vi "SinWaveGenerate 1.vi"() -> ()   [LabVIEW 2020]
uses:
  <vilib>/Utility/miscctls.llb/LVDateTimeRec.ctl
  <vilib>/Utility/miscctls.llb/LVAnnotationListTypeDef.ctl
  <vilib>/Waveform/WDTOps.llb/WDT Append Waveforms DBL.vi
  <vilib>/Waveform/WDTOps.llb/WDT Get Waveform Time Array DBL.vi
  <vilib>/measure/NI_MABase.lvlib
panel:
  in  "Kaydet":bool
  in  "Tabloları sil":bool
  in  "Oluştur":bool
  in  "Sinyaller arasını rampa ile birleştir":bool
  in  "Sin Fonksiyonları Arasındaki Düzeltme Artış Miktarı Amp":dbl=50.0 format="%#_13g"
  in  "Tab Control":T1(tab)
  out "Datada kullanılan sinyaller":waveform(dbl)[](graph)
  out "Sinyaller arasındaki geçiş kN farkı":cluster{i32[], "Y":dbl[]}[](graph)
  out "Sinyal Önizleme":waveform(dbl)(graph)
  out "Sinyal Önizleme":waveform(dbl)(graph)
  in  "stop":bool
  in  "Sin wave generate":T2(array[cluster])=[{"Örnekleme Ayarları"={"Fs"=100.0, "#s"=100.0}, "Sinyal Ayarları"={"Frekans"=1.0, "Faz"=0.0, "Genlik"=16.75, "Offset"=0.65, "Cycle"=6.0, "signal type"=enum."Sine Wave"}, "Amp Ratio"=1.0, "Toplam Tekrar"=1.0}, {"Örnekleme Ayarları"={"Fs"=100.0, "#s"=100.0}, "Sinyal Ayarları"={"Frekans"=1.0, "Faz"=0.0, "Genlik"=4.2, "Offset"=0.1, "Cycle"=1.0, "signal type"=enum."Sine Wave"}, "Amp Ratio"=1.0, "Toplam Tekrar"=9.0}, {"Örnekleme Ayarları"={"Fs"=100.0, "#s"=100.0}, "Sinyal Ayarları"={"Frekans"=1.0, "Faz"=0.0, "Genlik"=6.0, "Offset"=0.1, "Cycle"=1.0, "signal type"=enum."Sine Wave"}, "Amp Ratio"=1.0, "Toplam Tekrar"=50.0}, {"Örnekleme Ayarları"={"Fs"=100.0, "#s"=100.0}, "Sinyal Ayarları"={"Frekans"=1.0, "Faz"=0.0, "Genlik"=20.05, "Offset"=-7.45, "Cycle"=1.0, "signal type"=enum."Sine Wave"}, "Amp Ratio"=1.0, "Toplam Tekrar"=1.0}] {"Amp Ratio" format="%.2p"; "Sinyal Ayarları"."Faz" format="%.2p"; "Sinyal Ayarları"."Frekans" format="%0.2p"; "Örnekleme Ayarları"."Fs" format="%.2p"}
  # "Offset"
  # "Amplitude"
  # "Level 4"
  # "16,75"
  # "+0,65"
  # "Level 3"
  # "4,2"
  # "+0,1"
  # "Level 2"
  # "6,0"
  # "+0,1"
  # "Level 1"
  # "20,05"
  # "-7,45"
  # "array 0"
  # "array 1"
  # "array 2"
  # "array 3"
  # "((((((6xLevel 4)+level3)x9 )+ level2)x50)+ level1) x 200"
  # "(((Cycle*sinyal)*Toplam Tekrar + ......(Array n Cycle*Array n sinyal) * Array n Toplam Tekrar)))"
  # "Array 0 =>"
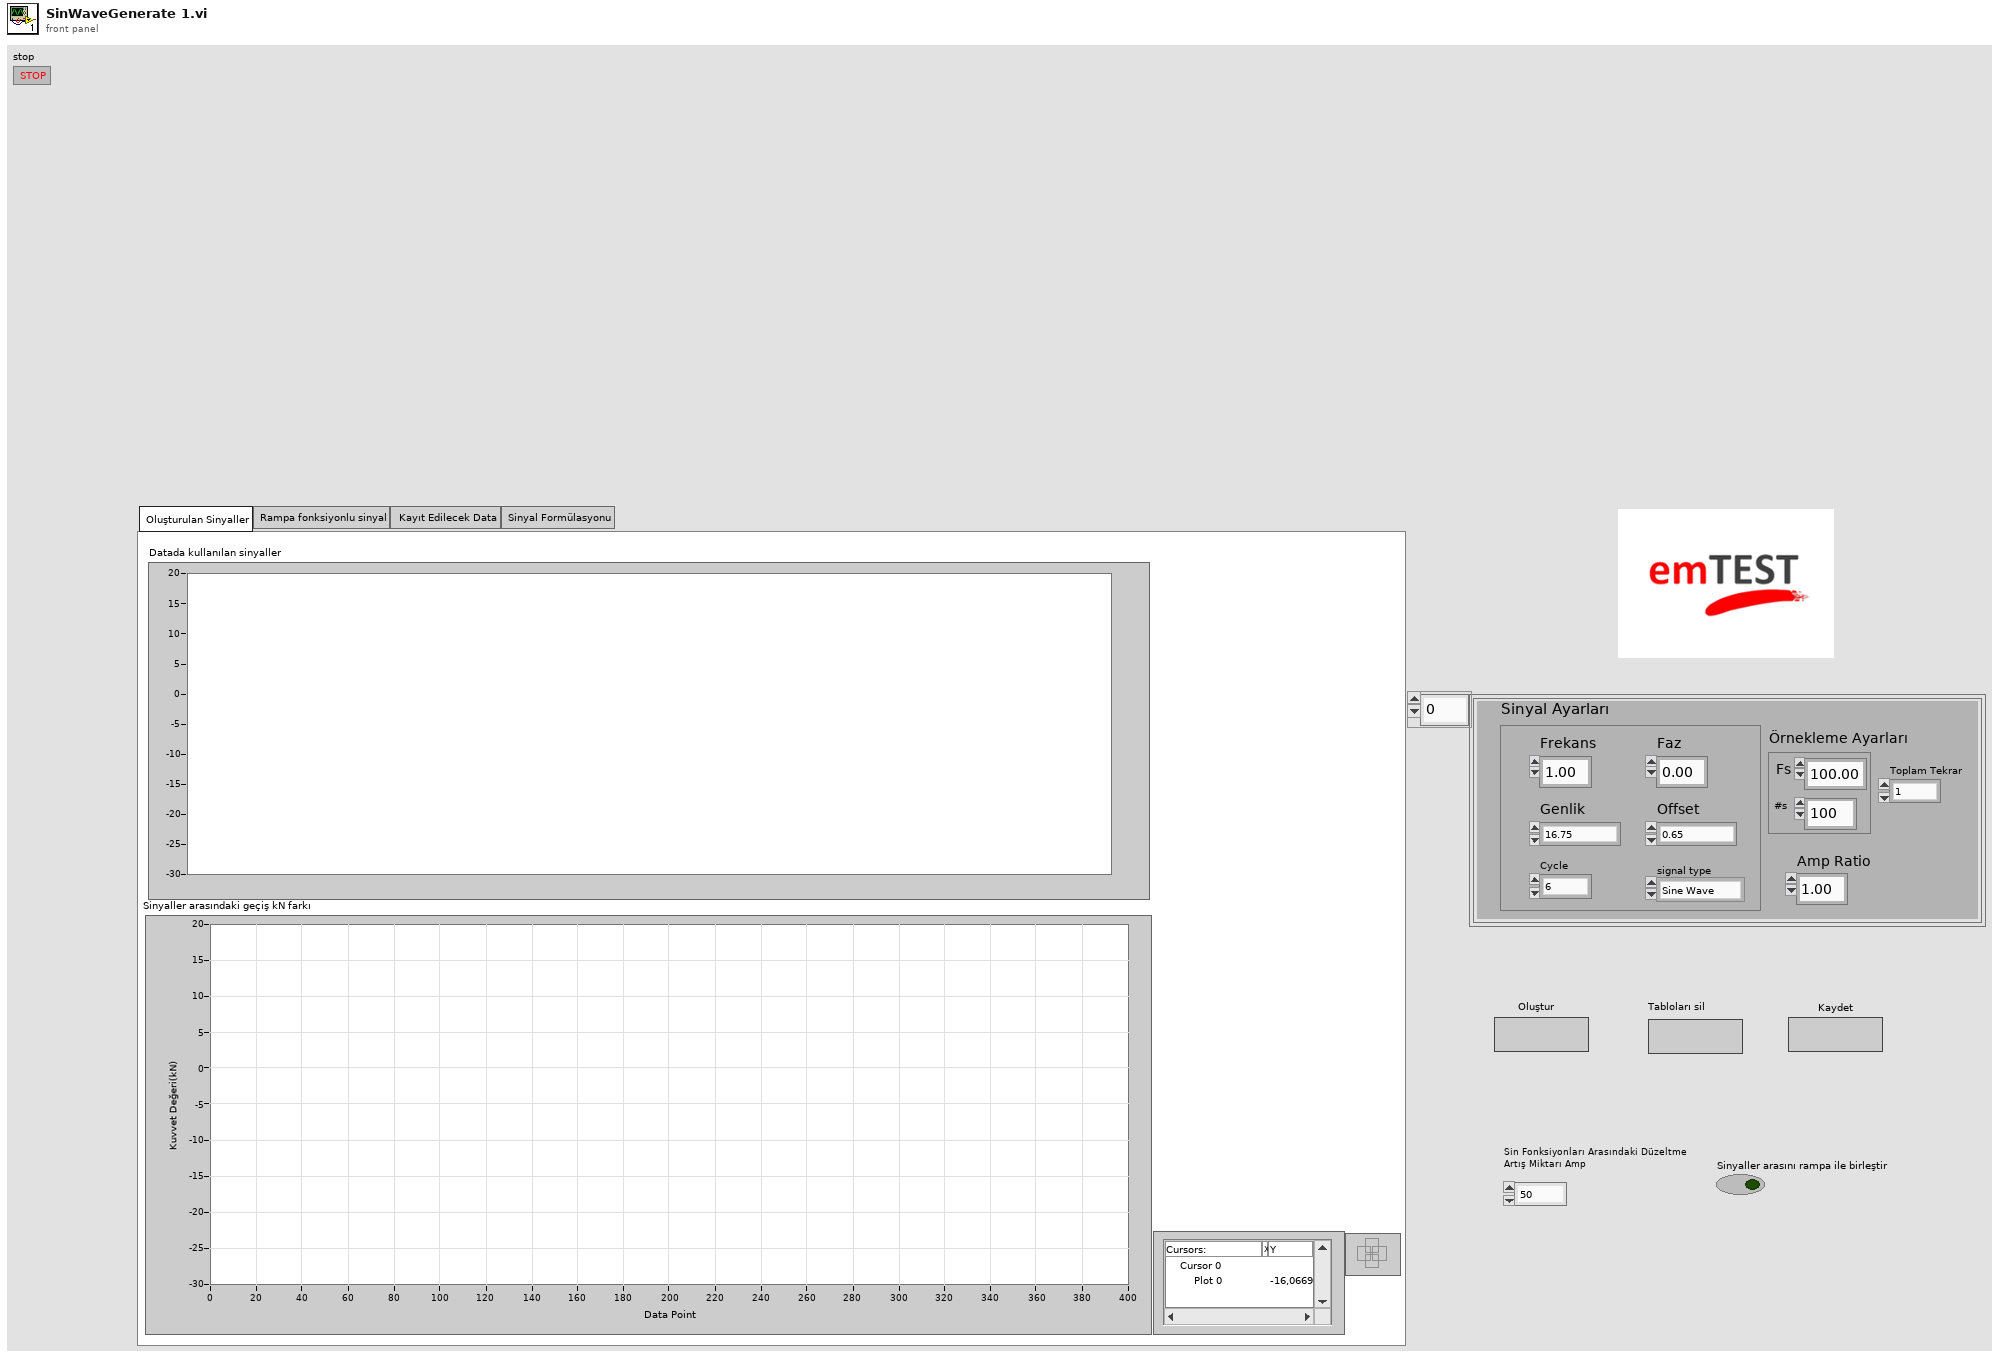
[diagram p1: front panel]
types:
  T1 = enum32{"Oluşturulan Sinyaller", "Rampa fonksiyonlu sinyal", "Kayıt Edilecek Data ", "Sinyal Formülasyonu"}
  T2 = cluster{"Örnekleme Ayarları":cluster{"Fs":dbl, "#s":dbl}, "Sinyal Ayarları":cluster{"Frekans":dbl, "Faz":dbl, "Genlik":dbl, "Offset":dbl, "Cycle":dbl, "signal type":enum16{"Sine Wave", "Triangle Wave", "Square Wave", "Sawtooth Wave"}}, "Amp Ratio":dbl, "Toplam Tekrar":dbl}[]
  T3 = enum16{"open", "replace", "create", "open or create", "replace or create", "replace or create with confirmation"}
  T4 = typedef "LVDateTimeRec.ctl" = cluster{"fractional second":dbl, "second":i32, "minute":i32, "hour":i32, "day of month":i32, "month":i32, "year":i32, "day of week":i32, "day of year":i32, "DST":i32}
  T5 = cluster{"Name":string, "Color":u32, "Style":u8, "Point Style":u8, "Name Visible":bool, "Allow Drag":bool, "Annotation Mode":u32, "Plot":i32, "Index":i32, "Position":cluster{"X":dbl, "Y":dbl}, "X Scale":u32, "Y Scale":u32, "Show Arrow":bool, "Lock Name":bool, "Plot Area":i32, "Label Offset":cluster{"X":dbl, "Y":dbl}}
  T6 = typedef "LVAnnotationListTypeDef.ctl" = cluster{"Name":string, "Color":u32, "Style":u8, "Point Style":u8, "Name Visible":bool, "Allow Drag":bool, "Annotation Mode":u32, "Plot":i32, "Index":i32, "Position":cluster{"X":dbl, "Y":dbl}, "X Scale":u32, "Y Scale":u32, "Show Arrow":bool, "Lock Name":bool, "Plot Area":i32, "Label Offset":cluster{"X":dbl, "Y":dbl}}[]
  T7 = enum16{"Sine Wave", "Triangle Wave", "Square Wave", "Sawtooth Wave"}
  T8 = cluster{"Frekans":dbl, "Faz":dbl, "Genlik":dbl, "Offset":dbl, "Cycle":dbl, "signal type":enum16{"Sine Wave", "Triangle Wave", "Square Wave", "Sawtooth Wave"}}
  T9 = cluster{"Name":string, "Color":u32, "Style":u8, "Point Style":u8, "Name Visible":bool, "Allow Drag":bool, "Annotation Mode":u32, "Plot":i32, "Index":i32, "Position":cluster{"X":dbl, "Y":dbl}, "X Scale":u32, "Y Scale":u32, "Show Arrow":bool, "Lock Name":bool, "Plot Area":i32, "Label Offset":cluster{"X":dbl, "Y":dbl}}[]
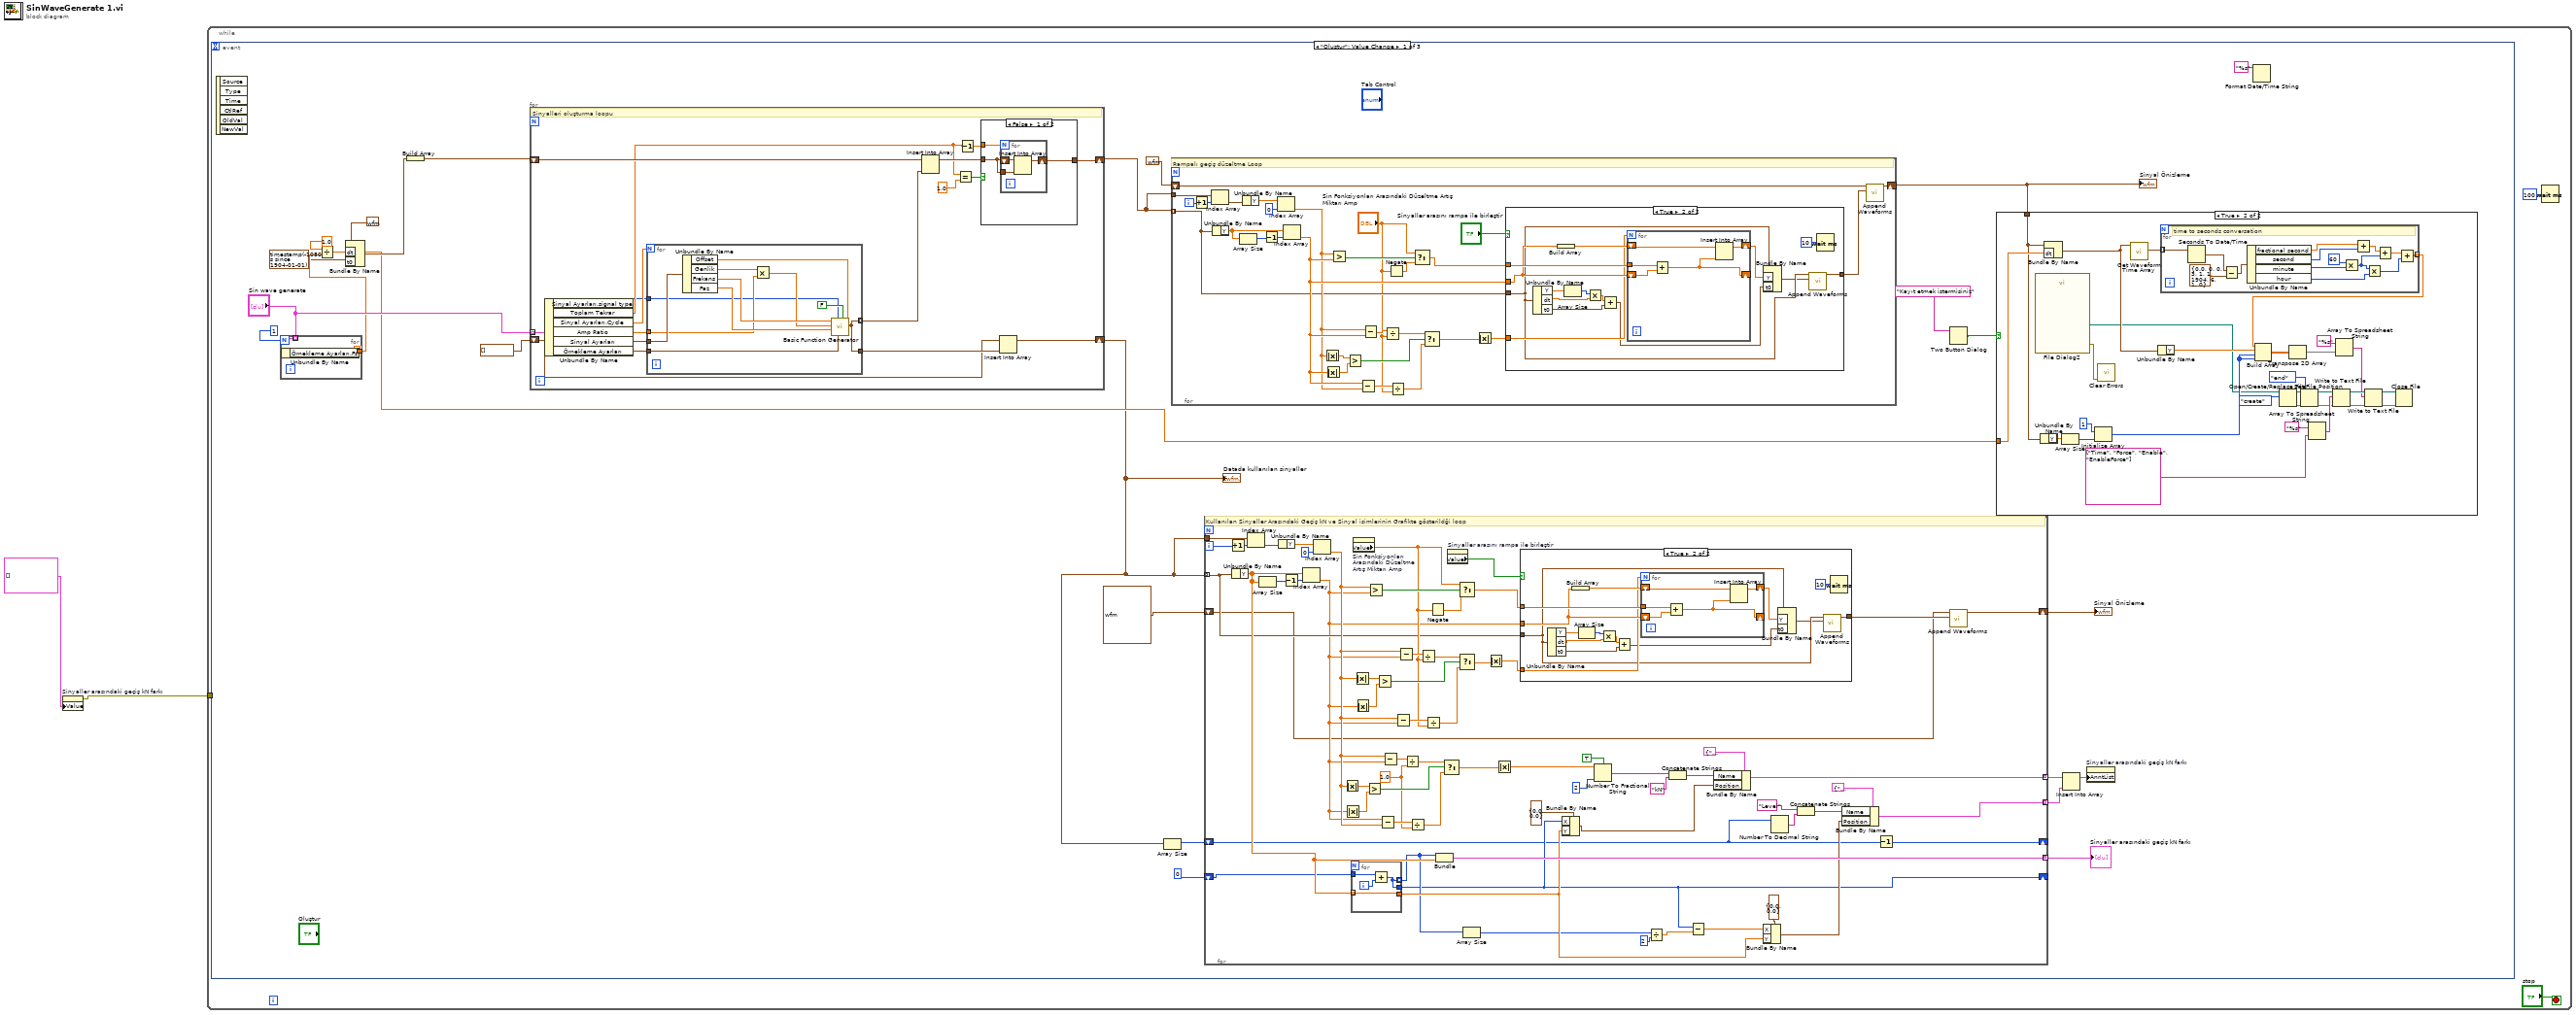
[diagram p0: block diagram]
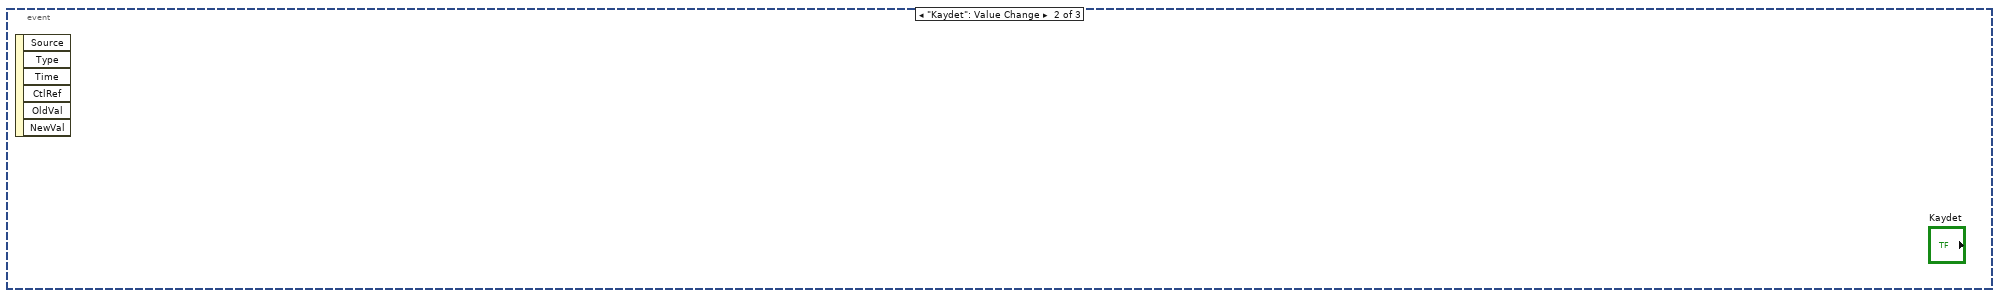
[diagram p6: hidden frame]
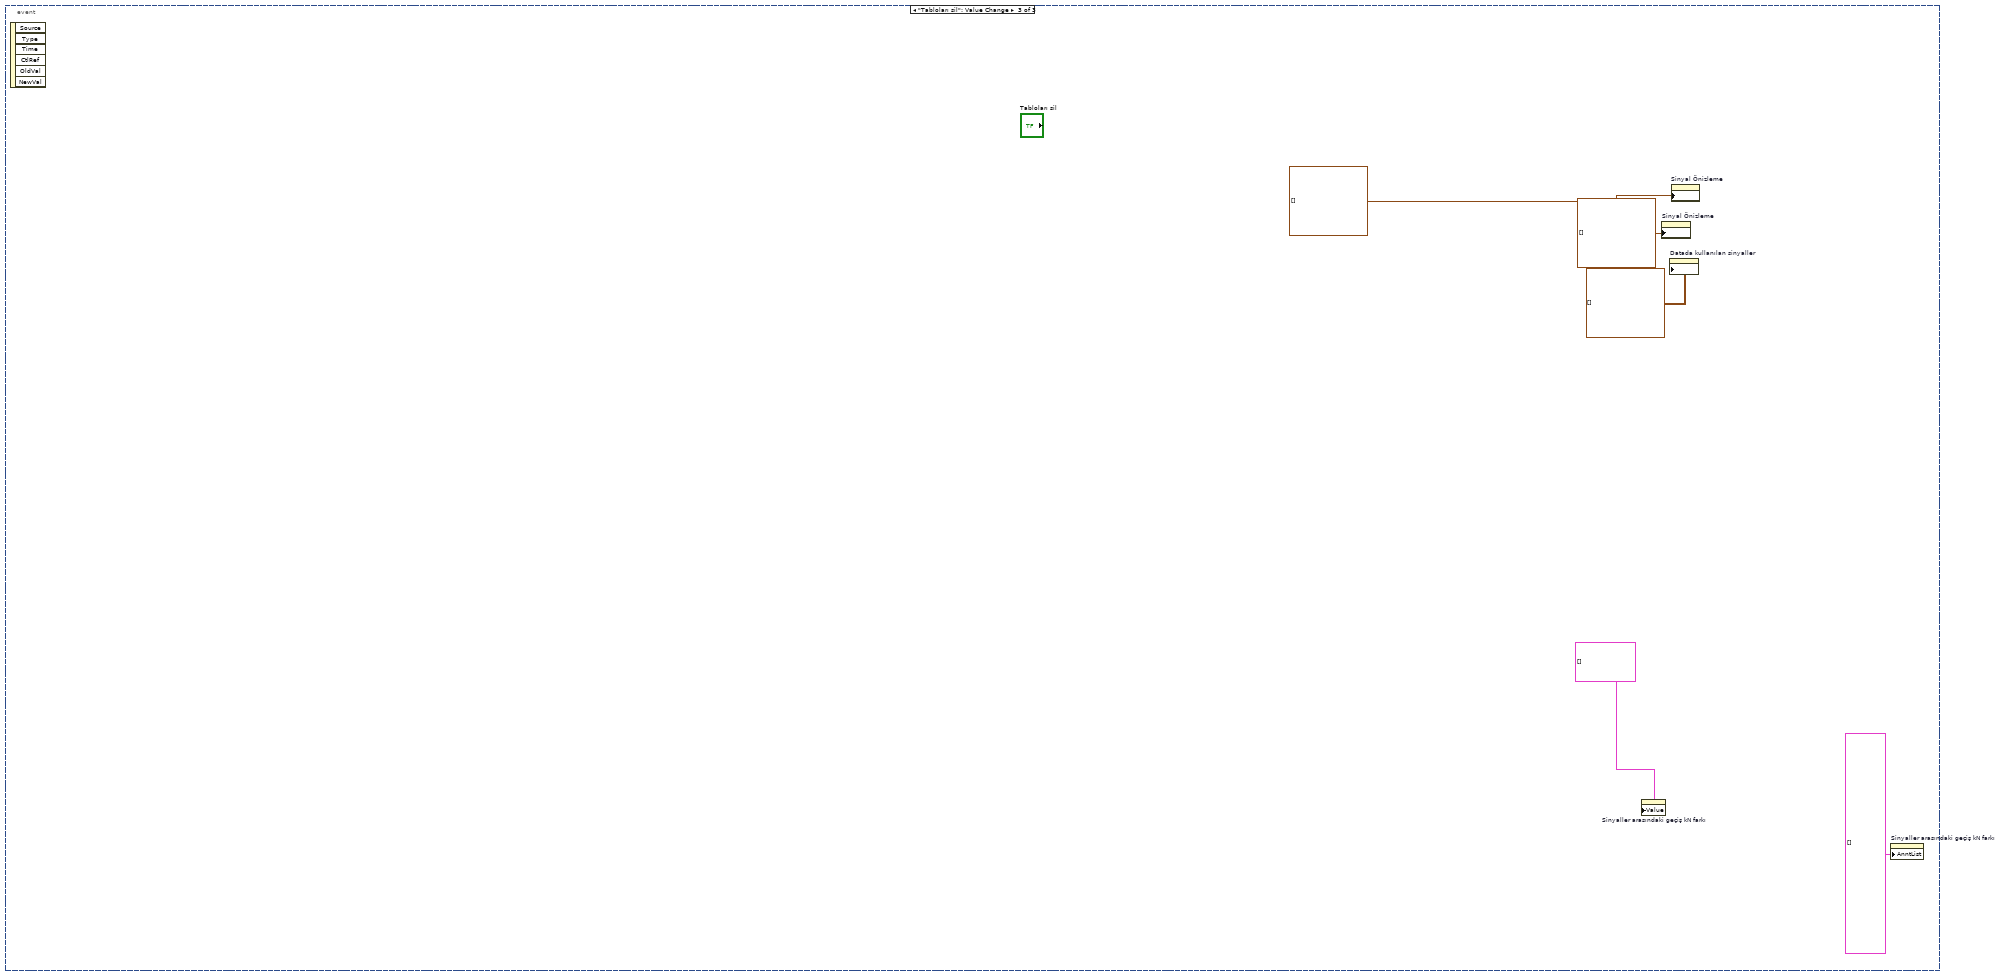
[diagram p7: hidden frame]
diagram:
  n1 = property on="Sinyaller arasındaki geçiş kN farkı" class="XYGraph (strict)"("Value"=cluster{i32[], "Y":dbl[]}[] [] ("XY Graph")) -> (error out=w1:errorcluster)  [unwired: 2 in, 1 out]
  n2 = while {
    tunnel: w1 -> [_]
    stop <- "stop" stop-if-true
    n3 = event shown="[0] \"Oluştur\": Value Change" {
      selector: _ -> [_ _ _]
      dyn-events: _ -> [_ _ _]
      timeout: _ -> [_ _ _]
      event "Oluştur": Value Change {
        n4 = event-data() -> ()  [unwired: 1 in, 6 out]
        n5 = for {
          N: 1 -> [_]
          tunnel: "Sin wave generate" -> [w215] mode=indexing
          tunnel: [w214] -> w25
          n6 = Unbundle By Name(w215) -> ("Örnekleme Ayarları.Fs"=w214:dbl)
        }
        n7 = Divide(x=1.0, y=w25) -> (x/y=w20:dbl)
        n8 = Bundle By Name(cluster=waveform(dbl) {"t0"=timestamp(0 s since 1904-01-01), "dt"=1.0, "Y"=[]} ("signal out"), "dt"=w20, "t0"=timestamp(-10800 s since 1904-01-01)) -> (w23:waveform(dbl))
        n9 = Build Array(w23) -> (w22:waveform(dbl)[])
        n10 = for {
          tunnel: "Sin wave generate" -> [w231] mode=indexing
          shift-right: [w224] -> w19
          shift-left: w22 -> [w230]
          shift-right: [w218] -> w6
          shift-left: waveform(dbl)[] [] -> [w217]
          # "Sinyalleri oluşturma loopu"
          n11 = Unbundle By Name(w231) -> ("Sinyal Ayarları.signal type"=w216:T7, "Toplam Tekrar"=w221:dbl, "Sinyal Ayarları.Cycle"=w227:dbl, "Amp Ratio"=w229:dbl, "Sinyal Ayarları"=w232:T8, "Örnekleme Ayarları"=w228:cluster{"Fs":dbl, "#s":dbl})
          n12 = for {
            N: w227 -> [_]
            tunnel: w232 -> [w248]
            tunnel: w229 -> [w246]
            tunnel: w228 -> [w243]
            tunnel: [w241] -> w226 mode=indexing
            tunnel: [w241] -> w219
            tunnel: w216 -> [w240]
            n13 = Unbundle By Name(w248) -> ("Offset"=w244:dbl, "Genlik"=w247:dbl, "Frekans"=w250:dbl, "Faz"=w249:dbl)
            n14 = Multiply(x=w247, y=w246) -> (x*y=w245:dbl)
            n15 = call <vilib>:"Basic Function Generator.vi"("offset"=w244, "reset signal"=FALSE, "sampling info"=w243, "signal type"=w240, "phase"=w249, "amplitude"=w245, "frequency"=w250) -> ("signal out"=w241:waveform(dbl))  [unwired: 2 in, 2 out]
          }
          n16 = Insert Into Array(array=w230, new element=w226) -> (w225:waveform(dbl)[])  [unwired: 1 in]
          n17 = Equal?(x=w221, y=1.0) -> (x = y?=w222:bool)
          n18 = Decrement(x=w221) -> (x-1=w220:dbl)
          n19 = case shown="False" w222 {
            tunnel: w225 -> [w235 w239]
            tunnel: w220 -> [w234 _]
            tunnel: [w233 w239] -> w224
            frame False {
              n20 = for {
                N: w234 -> [_]
                shift-right: [w237] -> w233
                shift-left: w235 -> [w238]
                tunnel: w235 -> [w236]
                n21 = Insert Into Array(array=w238, new element=w236) -> (w237:waveform(dbl)[])  [unwired: 1 in]
              }
            }
            frame True {
            }
          }
          n22 = Insert Into Array(array=w217, new element=w219) -> (w218:waveform(dbl)[])  [unwired: 1 in]
        }
        "Datada kullanılan sinyaller" <- w6
        n23 = Array Size(array=w6) -> (size(s)=w5:i32)
        n24 = for {
          tunnel: w19 -> [w170] mode=indexing
          tunnel: w19 -> [w189]
          shift-right: [w168] -> w14
          shift-left: waveform(dbl) {"t0"=timestamp(0 s since 1904-01-01), "dt"=1.0, "Y"=[]} ("waveform out") -> [w167]
          i -> [w188]
          # "Rampalı geçiş düzeltme Loop"
          n25 = Increment(x=w188) -> (x+1=w187:i32)
          n26 = Index Array(array=w189, index=w187) -> (element=w186:waveform(dbl))
          n27 = Unbundle By Name(w170) -> ("Y"=w190:dbl[])
          n28 = Array Size(array=w190) -> (size(s)=w191:i32)
          n29 = Unbundle By Name(w186) -> ("Y"=w185:dbl[])
          n30 = Decrement(x=w191) -> (x-1=w192:i32)
          n31 = Index Array(array=w185, index=0) -> (element=w175:dbl)
          n32 = Index Array(array=w190, index=w192) -> (element=w176:dbl)
          n33 = Absolute Value(x=w175) -> (abs(x)=w181:dbl)
          n34 = Absolute Value(x=w176) -> (abs(x)=w180:dbl)
          n35 = Greater?(x=w175, y=w176) -> (0:w182:bool)
          n36 = Greater?(x=w181, y=w180) -> (0:w179:bool)
          n37 = Subtract(x=w176, y=w175) -> (x-y=w174:dbl)
          n38 = Subtract(x=w175, y=w176) -> (x-y=w178:dbl)
          n39 = Divide(x=w178, y="Sin Fonksiyonları Arasındaki Düzeltme Artış Miktarı Amp") -> (x/y=w177:dbl)
          n40 = Negate(x="Sin Fonksiyonları Arasındaki Düzeltme Artış Miktarı Amp") -> (-x=w166:dbl)
          n41 = Divide(x=w174, y="Sin Fonksiyonları Arasındaki Düzeltme Artış Miktarı Amp") -> (x/y=w173:dbl)
          n42 = Select(t="Sin Fonksiyonları Arasındaki Düzeltme Artış Miktarı Amp", s=w182, f=w166) -> (s? t:f=w183:dbl)
          n43 = Select(t=w177, s=w179, f=w173) -> (s? t:f=w172:dbl)
          n44 = Absolute Value(x=w172) -> (abs(x)=w171:dbl)
          n45 = case shown="True" "Sinyaller arasını rampa ile birleştir" {
            tunnel: w170 -> [w193 w196]
            tunnel: w176 -> [_ w207]
            tunnel: w183 -> [_ w208]
            tunnel: [w193 w197] -> w169
            tunnel: w171 -> [_ w204]
            frame False {
            }
            frame True {
              n46 = Unbundle By Name(w196) -> ("Y"=w203:dbl[], "dt"=w198:dbl, "t0"=w200:timestamp)
              n47 = Build Array(w207) -> (w206:dbl[])
              n48 = Array Size(array=w203) -> (size(s)=w202:i32)
              n49 = Multiply(x=w202, y=w198) -> (x*y=w201:dbl)
              n50 = Add(x=w201, y=w200) -> (x+y=w199:timestamp)
              n51 = for {
                N: w204 -> [_]
                tunnel: w208 -> [w213]
                shift-right: [w209] -> _
                shift-left: w207 -> [w212]
                shift-right: [w211] -> w205
                shift-left: w206 -> [w210]
                n52 = Add(x=w213, y=w212) -> (x+y=w209:dbl)
                n53 = Insert Into Array(array=w210, new element=w209) -> (w211:dbl[])  [unwired: 1 in]
              }
              n54 = Bundle By Name(cluster=w196, "Y"=w205, "t0"=w199) -> (w195:waveform(dbl))
              n55 = call-poly <vilib>:"Append Waveforms.vi"("waveform B"=w195, "waveform A"=w196) -> ("waveform out"=w197:waveform(dbl))  [unwired: 8 in, 1 out]
              n56 = Wait (ms)(milliseconds to wait=u32 10) -> ()  [unwired: 1 out]
            }
          }
          n57 = call-poly <vilib>:"Append Waveforms.vi"("waveform B"=w169, "waveform A"=w167) -> ("waveform out"=w168:waveform(dbl))  [unwired: 8 in, 1 out]
        }
        "Sinyal Önizleme" <- w14
        n58 = for {
          tunnel: w6 -> [w100] mode=indexing
          tunnel: w6 -> [w136]
          shift-right: [w79] -> _
          shift-left: 0 -> [w76]
          tunnel: [w121] -> w17 mode=indexing
          tunnel: [w120] -> w9 mode=indexing
          shift-right: [w95] -> w16
          shift-left: waveform(dbl) {"t0"=timestamp(0 s since 1904-01-01), "dt"=1.0, "Y"=[]} -> [w94]
          tunnel: [w82] -> w8 mode=indexing
          shift-right: [w74] -> _
          shift-left: w5 -> [w73]
          i -> [w135]
          w119 = 1.0 ("y")
          # "Kullanılan Sinyaller Arasındaki Geçiş kN ve Sinyal isimlerinin Grafikte gösterildği loop"
          n59 = Increment(x=w135) -> (x+1=w134:i32)
          n60 = Unbundle By Name(w100) -> ("Y"=w122:dbl[])
          n61 = Index Array(array=w136, index=w134) -> (element=w133:waveform(dbl))
          n62 = Array Size(array=w122) -> (size(s)=w137:i32)
          n63 = Unbundle By Name(w133) -> ("Y"=w132:dbl[])
          n64 = Decrement(x=w137) -> (x-1=w138:i32)
          n65 = Index Array(array=w122, index=w138) -> (element=w99:dbl)
          n66 = Index Array(array=w132, index=0) -> (element=w104:dbl)
          n67 = Absolute Value(x=w104) -> (abs(x)=w130:dbl)
          n68 = Absolute Value(x=w99) -> (abs(x)=w129:dbl)
          n69 = for {
            tunnel: w122 -> [w160] mode=indexing
            tunnel: [w162] -> w81 mode=indexing
            tunnel: [w162] -> w79
            tunnel: w76 -> [w161]
            tunnel: [w160] -> w84
            i -> [w163]
            n70 = Add(x=w161, y=w163) -> (x+y=w162:i32)
          }
          n71 = property on="Sin Fonksiyonları Arasındaki Düzeltme Artış Miktarı Amp" class="DigNum (strict)"() -> ("Value"=w103:dbl)  [unwired: 2 in, 2 out]
          n72 = Absolute Value(x=w104) -> (abs(x)=w105:dbl)
          n73 = Absolute Value(x=w99) -> (abs(x)=w106:dbl)
          n74 = Greater?(x=w130, y=w129) -> (0:w128:bool)
          n75 = Greater?(x=w104, y=w99) -> (0:w113:bool)
          n76 = Greater?(x=w105, y=w106) -> (0:w107:bool)
          n77 = Subtract(x=w99, y=w104) -> (x-y=w125:dbl)
          n78 = Subtract(x=w104, y=w99) -> (x-y=w127:dbl)
          n79 = Subtract(x=w104, y=w99) -> (x-y=w110:dbl)
          n80 = Subtract(x=w104, y=w99) -> (x-y=w108:dbl)
          n81 = Divide(x=w127, y=w119) -> (x/y=w126:dbl)
          n82 = Divide(x=w125, y=w119) -> (x/y=w124:dbl)
          n83 = Divide(x=w108, y=w103) -> (x/y=w109:dbl)
          n84 = Divide(x=w110, y=w103) -> (x/y=w111:dbl)
          n85 = Negate(x=w103) -> (-x=w112:dbl)
          n86 = Bundle(w81, "Y"=w122) -> (w121:cluster{i32[], "Y":dbl[]})  [unwired: 1 in]
          n87 = Select(t=w126, s=w128, f=w124) -> (s? t:f=w123:dbl)
          n88 = property on="Sinyaller arasını rampa ile birleştir" class="Bool (strict)"() -> ("Value"=w102:bool)  [unwired: 2 in, 2 out]
          n89 = Select(t=w103, s=w113, f=w112) -> (s? t:f=w101:dbl)
          n90 = Select(t=w109, s=w107, f=w111) -> (s? t:f=w98:dbl)
          n91 = Array Size(array=w81) -> (size(s)=w80:i32)
          n92 = Absolute Value(x=w98) -> (abs(x)=w97:dbl)
          n93 = Absolute Value(x=w123) -> (abs(x)=w116:dbl)
          n94 = case shown="True" w102 {
            tunnel: w100 -> [w139 w142]
            tunnel: w99 -> [_ w153]
            tunnel: w101 -> [_ w154]
            tunnel: [w139 w143] -> w96
            tunnel: w97 -> [_ w150]
            frame False {
            }
            frame True {
              n95 = Unbundle By Name(w142) -> ("Y"=w149:dbl[], "dt"=w144:dbl, "t0"=w146:timestamp)
              n96 = Build Array(w153) -> (w152:dbl[])
              n97 = Array Size(array=w149) -> (size(s)=w148:i32)
              n98 = Multiply(x=w148, y=w144) -> (x*y=w147:dbl)
              n99 = Add(x=w147, y=w146) -> (x+y=w145:timestamp)
              n100 = for {
                N: w150 -> [_]
                tunnel: w154 -> [w159]
                shift-right: [w155] -> _
                shift-left: w153 -> [w158]
                shift-right: [w157] -> w151
                shift-left: w152 -> [w156]
                n101 = Add(x=w159, y=w158) -> (x+y=w155:dbl)
                n102 = Insert Into Array(array=w156, new element=w155) -> (w157:dbl[])  [unwired: 1 in]
              }
              n103 = Bundle By Name(cluster=w142, "Y"=w151, "t0"=w145) -> (w141:waveform(dbl))
              n104 = call-poly <vilib>:"Append Waveforms.vi"("waveform B"=w141, "waveform A"=w142) -> ("waveform out"=w143:waveform(dbl))  [unwired: 8 in, 1 out]
              n105 = Wait (ms)(milliseconds to wait=u32 10) -> ()  [unwired: 1 out]
            }
          }
          n106 = Bundle By Name(cluster=cluster{"X":dbl, "Y":dbl} {"X"=0.0, "Y"=0.0} ("Position"), "X"=w79, "Y"=w84) -> (w114:cluster{"X":dbl, "Y":dbl})
          n107 = Number To Fractional String(use system decimal point (T)=TRUE, number=w116, precision (6)=i16 2) -> (F-format string=w90:string)  [unwired: 1 in]
          n108 = Divide(x=w80, y=2) -> (x/y=w78:dbl)
          n109 = Concatenate Strings(w90, "kN" ("string")) -> (w91:string)
          n110 = Subtract(x=w79, y=w78) -> (x-y=w77:dbl)
          n111 = Bundle By Name(cluster=T5 {"Name"="Note0", "Color"=10, "Style"=0, "Point Style"=0, "Name Visible"=TRUE, "Allow Drag"=TRUE, "Annotation Mode"=0, "Plot"=0, "Index"=0, "Position"={"X"=0.0, "Y"=0.0}, "X Scale"=0, "Y Scale"=0, "Show Arrow"=TRUE, "Lock Name"=FALSE, "Plot Area"=0, "Label Offset"={"X"=0.0, "Y"=0.0}}, "Name"=w91, "Position"=w114) -> (w120:T5)
          n112 = Bundle By Name(cluster=cluster{"X":dbl, "Y":dbl} {"X"=0.0, "Y"=0.0} ("Position"), "X"=w77, "Y"=w84) -> (w85:cluster{"X":dbl, "Y":dbl})
          n113 = Number To Decimal String(number=w73) -> (decimal integer string=w75:string)  [unwired: 1 in]
          n114 = Concatenate Strings("Level" ("string"), w75) -> (w89:string)
          n115 = Bundle By Name(cluster=T5 {"Name"="Note0", "Color"=10, "Style"=0, "Point Style"=0, "Name Visible"=TRUE, "Allow Drag"=TRUE, "Annotation Mode"=0, "Plot"=0, "Index"=0, "Position"={"X"=0.0, "Y"=0.0}, "X Scale"=0, "Y Scale"=0, "Show Arrow"=TRUE, "Lock Name"=FALSE, "Plot Area"=0, "Label Offset"={"X"=0.0, "Y"=0.0}}, "Name"=w89, "Position"=w85) -> (w82:T5)
          n116 = Decrement(x=w73) -> (x-1=w74:i32)
          n117 = call-poly <vilib>:"Append Waveforms.vi"("waveform B"=w96, "waveform A"=w94) -> ("waveform out"=w95:waveform(dbl))  [unwired: 8 in, 1 out]
        }
        "Sinyal Önizleme" <- w16
        "Sinyaller arasındaki geçiş kN farkı" <- w17
        n118 = Two Button Dialog(message="Kayıt etmek istermisiniz") -> (T button?=w12:bool)  [unwired: 2 in]
        n119 = case shown="True" w12 {
          tunnel: w20 -> [_ w58]
          tunnel: w14 -> [_ w53]
          frame False {
          }
          frame True {
            n120 = call "File Dialog2"() -> ("selected path"=w47:path, "error out"=w57:errorcluster)  [unwired: 12 in, 2 out]
            n121 = Unbundle By Name(w53) -> ("Y"=w56:dbl[])
            n122 = Bundle By Name(cluster=w53, "dt"=w58) -> (w52:waveform(dbl))
            n123 = Array Size(array=w56) -> (size(s)=w55:i32)
            n124 = Initialize Array(i16 1 ("element"), w55) -> (w48:i16[])
            n125 = call <vilib>:"Clear Errors.vi"("error in (no error)"=w57) -> ()  [unwired: 5 in, 2 out]
            n126 = call-poly <vilib>:"Get Waveform Time Array.vi"("waveform in"=w52) -> ("X array"=w50:timestamp[])  [unwired: 9 in, 1 out]
            n127 = Unbundle By Name(w52) -> ("Y"=w51:dbl[])
            n128 = for {
              tunnel: w50 -> [w72] mode=indexing
              tunnel: [w63] -> w49 mode=indexing
              # "time to seconds conversation"
              n129 = Seconds To Date/Time(time stamp (now)=w72) -> (date time rec=w71:T4)  [unwired: 1 in]
              n130 = Subtract(x=w71, y=T4 {"fractional second"=0.0, "second"=0, "minute"=0, "hour"=3, "day of month"=1, "month"=1, "year"=1904, "day of week"=6, "day of year"=1, "DST"=0} ("date time rec")) -> (x-y=w69:T4)
              n131 = Unbundle By Name(w69) -> ("fractional second"=w68:dbl, "second"=w67:i32, "minute"=w65:i32, "hour"=w64:i32)
              n132 = Multiply(x=i16 60, y=w65) -> (x*y=w61:i32)
              n133 = Add(x=w68, y=w67) -> (x+y=w62:dbl)
              n134 = Multiply(x=w61, y=w64) -> (x*y=w59:i32)
              n135 = Add(x=w62, y=w61) -> (x+y=w60:dbl)
              n136 = Add(x=w60, y=w59) -> (x+y=w63:dbl)
            }
            n137 = Build Array(w49, w51, w48, w48) -> (w32:dbl[][])
            n138 = Open/Create/Replace File(file path (use dialog)=w47, operation (0:open)=T3."create") -> (refnum out=w45:refnum<file>, error out=w39:errorcluster)  [unwired: 4 in, 1 out]
            n139 = Transpose 2D Array(2D array=w32) -> (transposed array=w31:dbl[][])
            n140 = Set File Position(refnum=w45, from (0:start)=enum16{"start", "end", "current"}."end", error in=w39) -> (refnum out=w43:refnum<file>, error out=w40:errorcluster)  [unwired: 1 in]
            n141 = Array To Spreadsheet String(array=string[] ["Time", "Force", "Enable", "EnableForce"], 3:"%s" ("delimiter (Tab)")) -> (spreadsheet string=w42:string)  [unwired: 1 in]
            n142 = Write to Text File(file (use dialog)=w43, text=w42, error in=w40) -> (refnum out=w37:refnum<file>, error out=w36:errorcluster)  [unwired: 1 in, 1 out]
            n143 = Array To Spreadsheet String(array=w31, 3:"%s" ("delimiter (Tab)")) -> (spreadsheet string=w33:string)  [unwired: 1 in]
            n144 = Write to Text File(file (use dialog)=w37, text=w33, error in=w36) -> (refnum out=w35:refnum<file>, error out=w34:errorcluster)  [unwired: 1 in, 1 out]
            n145 = Close File(refnum=w35, error in=w34) -> ()  [unwired: 2 out]
          }
        }
        n146 = Insert Into Array(array=w9, new element=w8) -> (w7:T9)  [unwired: 1 in]
        n147 = property on="Sinyaller arasındaki geçiş kN farkı" class="XYGraph (strict)"("AnntList"=w7) -> ()  [unwired: 2 in, 2 out]
        n148 = Format Date/Time String(time format string (%c)="%s") -> ()  [unwired: 2 in, 1 out]
      }
      event "Kaydet": Value Change {
        n149 = event-data() -> ()  [unwired: 1 in, 6 out]
      }
      event "Tabloları sil": Value Change {
        n150 = event-data() -> ()  [unwired: 1 in, 6 out]
        n151 = property on="Sinyaller arasındaki geçiş kN farkı" class="XYGraph (strict)"("Value"=cluster{i32[], "Y":dbl[]}[] [] ("XY Graph")) -> ()  [unwired: 2 in, 2 out]
        n152 = property on="Sinyal Önizleme" class="WFChart (strict)"("History Data"=waveform(dbl)[] []) -> ()  [unwired: 2 in, 2 out]
        n153 = property on="Datada kullanılan sinyaller" class="WFChart (strict)"("History Data"=waveform(dbl)[][] []) -> ()  [unwired: 2 in, 2 out]
        n154 = property on="Sinyal Önizleme" class="WFChart (strict)"("History Data"=waveform(dbl)[] []) -> ()  [unwired: 2 in, 2 out]
        n155 = property on="Sinyaller arasındaki geçiş kN farkı" class="XYGraph (strict)"("AnntList"=T6 [] ("Annotation List")) -> ()  [unwired: 2 in, 2 out]
      }
    }
    n156 = Wait (ms)(milliseconds to wait=u32 100) -> ()  [unwired: 1 out]
  }
